vi "Gyroscope Correct.vi"(2 "Check":dbl, 4 "YAW":dbl) -> (0 "Out motor":dbl, 1 "Ok":bool)   [LabVIEW 2020]
panel:
  out "coerced(x)":dbl
  out "check - motor":bool
  out "yaw - motor":bool
  out "yaw - check":bool
  out "Rez":dbl
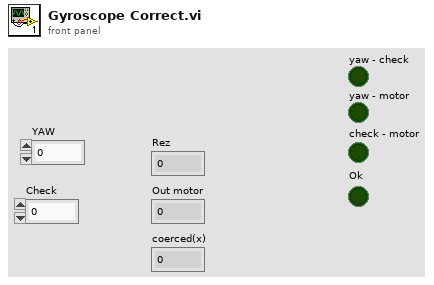
[diagram p1: front panel]
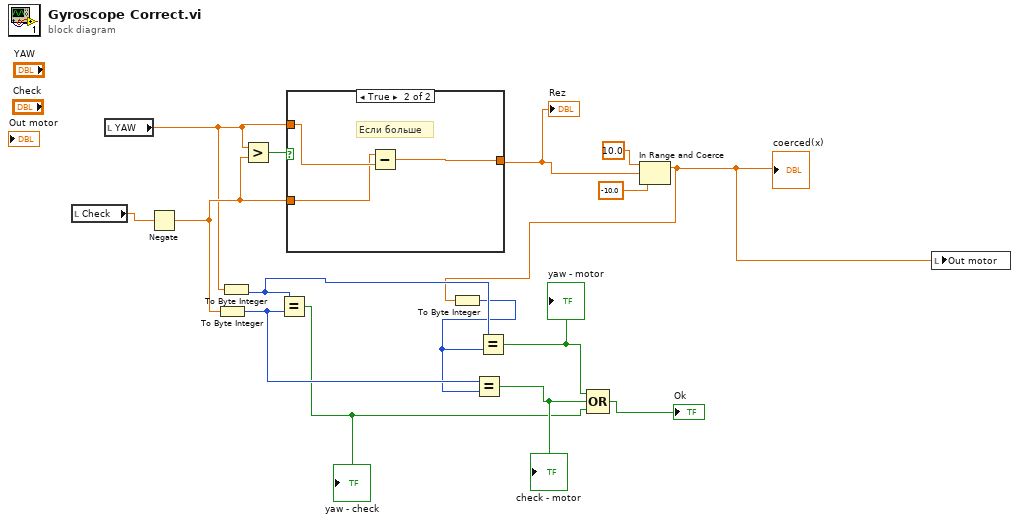
[diagram p0: block diagram]
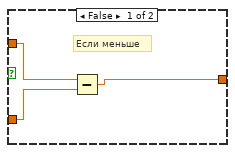
[diagram p2: hidden frame]
diagram:
  n1 = local read "Check"() -> (w7:dbl)
  n2 = local read "YAW"() -> (w4:dbl)
  n3 = Negate(x=w7) -> (-x=w5:dbl)
  n4 = To Byte Integer(number=w5) -> (8bit integer=w11:i8)
  n5 = To Byte Integer(number=w4) -> (8bit integer=w12:i8)
  n6 = Greater?(x=w4, y=w5) -> (0:w15:bool)
  n7 = Equal?(x=w12, y=w11) -> (x = y?=w3:bool)
  "yaw - check" <- w3
  n8 = case shown="True" w15 {
    tunnel: w4 -> [w17 w20]
    tunnel: w5 -> [w16 w19]
    tunnel: [w18 w21] -> w6
    frame False {
      # "Если меньше"
      n9 = Subtract(x=w17, y=w16) -> (x-y=w18:dbl)
    }
    frame True {
      # "Если больше"
      n10 = Subtract(x=w19, y=w20) -> (x-y=w21:dbl)
    }
  }
  "Rez" <- w6
  n11 = In Range and Coerce(upper limit=10.0, x=w6, lower limit=-10.0) -> (coerced(x)=w1:dbl)  [unwired: 1 out]
  "coerced(x)" <- w1
  n12 = To Byte Integer(number=w1) -> (8bit integer=w10:i8)
  n13 = Equal?(x=w11, y=w10) -> (x = y?=w8:bool)
  "check - motor" <- w8
  n14 = Equal?(x=w12, y=w10) -> (x = y?=w9:bool)
  "yaw - motor" <- w9
  n15 = Compound Arithmetic op=OR(w9, w8, w3) -> (→"Ok":bool)
  n16 = local write "Out motor"(w1) -> ()
